vi "SetMotionDelay.vi"(1 "Motor Speed":u16(ring)=65000 items=["SLOW"=3300, "MEDIUM"=30000, "FAST"=65000], 2 "XY Vector":dbl[](array[numeric])) -> (0 "Delays":dbl[](array[numeric]))   [LabVIEW 2015]
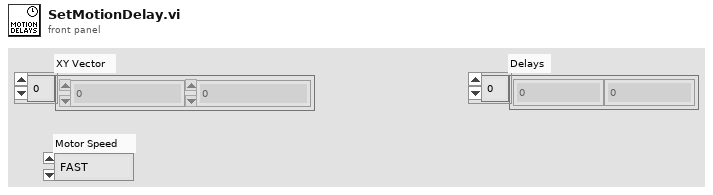
[diagram p1: front panel]
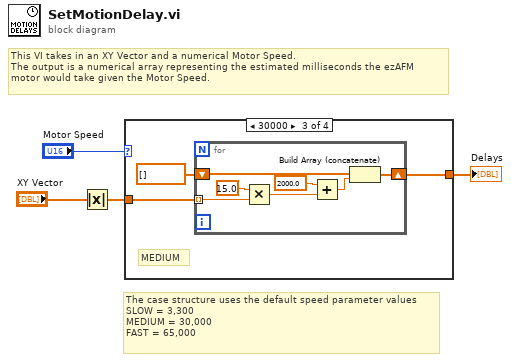
[diagram p0: block diagram]
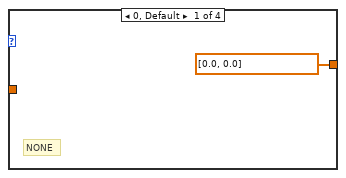
[diagram p2: hidden frame]
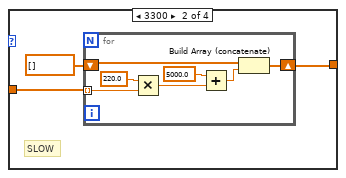
[diagram p3: hidden frame]
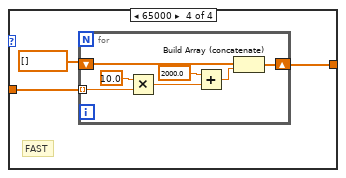
[diagram p4: hidden frame]
diagram:
  # "The case structure uses the default speed parameter values \nSLOW = 3,300\nMEDIUM = 30,000\nFAST = 65,000"
  # "This VI takes in an XY Vector and a numerical Motor Speed.\nThe output is a numerical array representing the estimated milliseconds the ezAFM\nmotor would take given the Motor Speed."
  n1 = Absolute Value(x="XY Vector") -> (abs(x)=w1:dbl[])
  n2 = case shown="30000" "Motor Speed" {
    tunnel: w1 -> [_ w7 w18 w28]
    tunnel: [dbl[] [0.0, 0.0] w8 w17 w27] -> w4
    frame 0, Default {
      # "NONE"
    }
    frame 3300 {
      # "SLOW"
      n3 = for {
        tunnel: w7 -> [w15] mode=indexing
        shift-right: [w10] -> w8
        shift-left: dbl[] [] -> [w9]
        n4 = Multiply(x=220.0, y=w15) -> (x*y=w12:dbl)
        n5 = Add(x=5000.0, y=w12) -> (x+y=w11:dbl)
        n6 = Build Array (concatenate)(w9, w11) -> (w10:dbl[])
      }
    }
    frame 30000 {
      # "MEDIUM"
      n7 = for {
        tunnel: w18 -> [w25] mode=indexing
        shift-right: [w20] -> w17
        shift-left: dbl[] [] -> [w19]
        n8 = Multiply(x=15.0, y=w25) -> (x*y=w22:dbl)
        n9 = Add(x=2000.0, y=w22) -> (x+y=w21:dbl)
        n10 = Build Array (concatenate)(w19, w21) -> (w20:dbl[])
      }
    }
    frame 65000 {
      # "FAST"
      n11 = for {
        tunnel: w28 -> [w35] mode=indexing
        shift-right: [w30] -> w27
        shift-left: dbl[] [] -> [w29]
        n12 = Multiply(x=10.0, y=w35) -> (x*y=w32:dbl)
        n13 = Add(x=2000.0, y=w32) -> (x+y=w31:dbl)
        n14 = Build Array (concatenate)(w29, w31) -> (w30:dbl[])
      }
    }
  }
  "Delays" <- w4
